vi "LJM logger read program config.vi"(4 "filename":string="expconfig.cfg", 5 "Working Directory":path) -> (0 "error out":errorcluster, 1 "Good Program Config":bool, 2 "Program Configs Out":T1={"Data File Prefix"="", "Scan Rate (Hz)"=0.0, "Graph History"=0, "# Channels"=0, "Disable Scaling"=FALSE, "Max File Size (Bytes)"=0, "Channel Setup"={"Name"=["AIN0", "AIN1", "AIN2", "AIN3", "AIN4", "AIN5", "AIN6", "AIN7", "AIN8", "AIN9", "AIN10", "AIN11", "AIN12", "AIN13", "AIN14", "AIN15"], "", "Scaling Equation"=["y=a", "y=b", "y=c", "y=d", "y=e", "y=f", "y=g", "y=h", "y=i", "y=j", "y=k", "y=l", "y=m", "y=n", "y=o", "y=p"], "", "Graph?"=[TRUE, TRUE, TRUE, TRUE, FALSE, FALSE, FALSE, FALSE, FALSE, FALSE, FALSE, FALSE, FALSE, FALSE, FALSE, FALSE]}, "Interval (ms)"=0, "Write To File"=FALSE, "Log Every n Scans"=0})   [LabVIEW 2026]
uses:
  Common Logger Controls/Program Config Cluster.ctl
  Common Logger Controls/Channel Setup.ctl
  <vilib>/Utility/config.llb/Read Key (String).vi
  <vilib>/Utility/config.llb/Read Key (I32).vi
  <vilib>/Utility/config.llb/Read Key (U32).vi
  <vilib>/Utility/config.llb/Read Key (Double).vi
  <vilib>/Utility/config.llb/Read Key (Boolean).vi
  <vilib>/Utility/config.llb/NI_LVConfig.lvlib
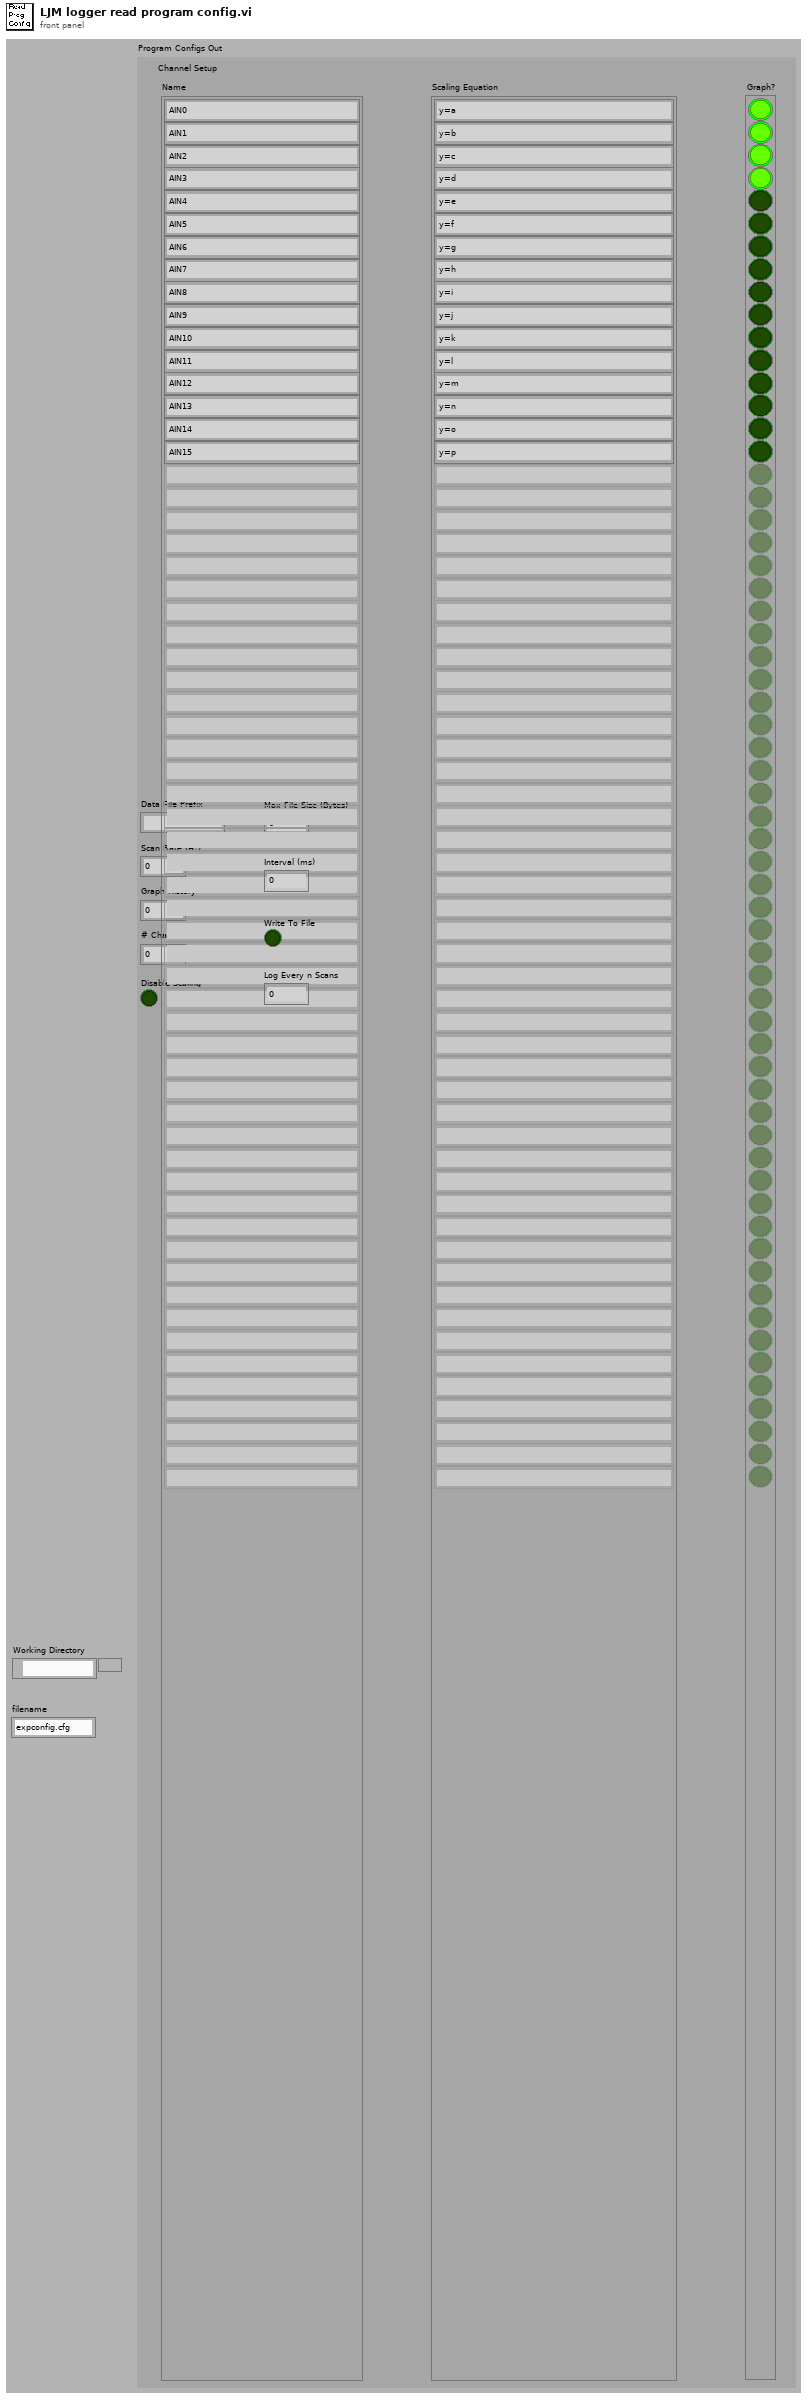
[diagram p1: front panel]
types:
  T1 = typedef "Program Config Cluster.ctl" = cluster{"Data File Prefix":string, "Scan Rate (Hz)":dbl, "Graph History":i32, "# Channels":i32, "Disable Scaling":bool, "Max File Size (Bytes)":i32, "Channel Setup":T2, "Interval (ms)":u32, "Write To File":bool, "Log Every n Scans":i32}
  T2 = typedef "Channel Setup.ctl" = cluster{"Name":string[], string, "Scaling Equation":string[], string, "Graph?":bool[]}
  T3 = typedef "NI_LVConfig.lvlib/Config Data RefNum.ctl" = refnum<k1>
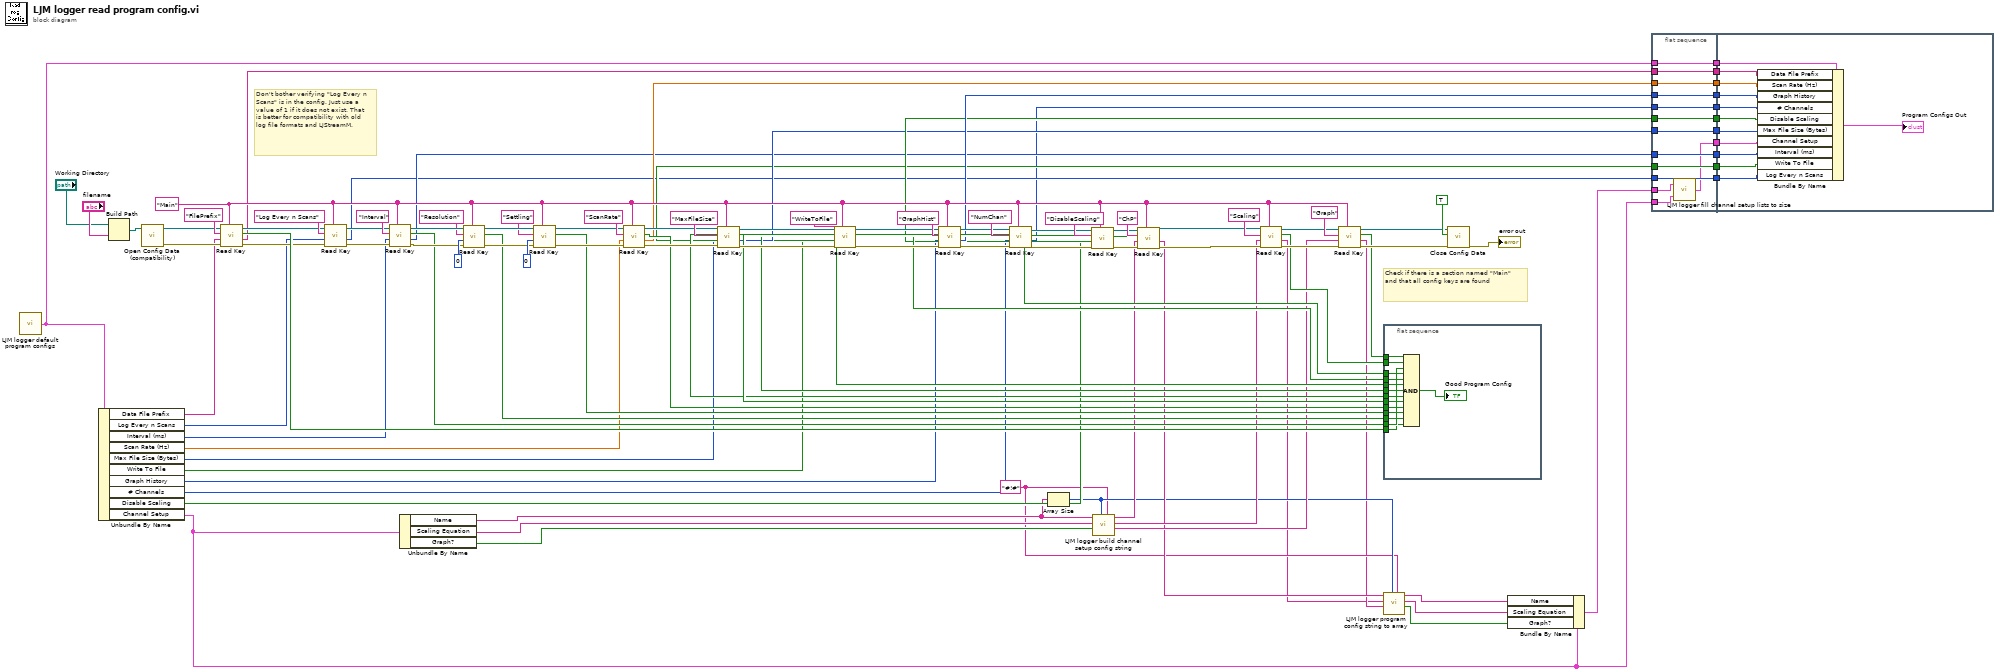
[diagram p0: block diagram]
diagram:
  w6 = "#!#" ("delimiter (#!#)")
  w54 = "Main" ("section")
  # "Don't bother verifying \"Log Every n Scans\" is in the config. Just use a value of 1 if it does not exist. That is better for compatibility with old log file formats and LJStreamM."
  # "Check if there is a section named \"Main\" and that all config keys are found"
  n1 = call "LJM logger default program configs.vi"() -> ("Program Configs"=w10:T1)  [unwired: 1 in]
  n2 = Unbundle By Name(w10) -> ("Data File Prefix"=w35:string, "Log Every n Scans"=w34:i32, "Interval (ms)"=w33:u32, "Scan Rate (Hz)"=w32:dbl, "Max File Size (Bytes)"=w31:i32, "Write To File"=w30:bool, "Graph History"=w29:i32, "# Channels"=w8:i32, "Disable Scaling"=w28:bool, "Channel Setup"=w1:T2)
  n3 = Build Path(base path="Working Directory", name or relative path="filename") -> (appended path=w110:path)
  n4 = call <vilib>:"Open Config Data (compatibility).vi"("configuration file path"=w110) -> ("error out"=w56:errorcluster, "refnum"=w57:T3)  [unwired: 8 in, 1 out]
  n5 = call-poly <vilib>:"Read Key.vi"("section"=w54, "error in (no error)"=w56, "default value"=w35, "key"="FilePrefix", "refnum"=w57) -> ("error out"=w53:errorcluster, "value"=w48:string, "found?"=w69:bool, "refnum out"=w51:T3)  [unwired: 3 in]
  n6 = call-poly <vilib>:"Read Key.vi"("section"=w54, "error in (no error)"=w53, "default value"=w34, "key"="Log Every n Scans", "refnum"=w51) -> ("error out"=w52:errorcluster, "value"=w41:i32, "refnum out"=w50:T3)  [unwired: 3 in, 1 out]
  n7 = call-poly <vilib>:"Read Key.vi"("section"=w54, "error in (no error)"=w52, "default value"=w33, "key"="Interval", "refnum"=w50) -> ("error out"=w85:errorcluster, "value"=w43:u32, "found?"=w68:bool, "refnum out"=w84:T3)  [unwired: 3 in]
  n8 = Unbundle By Name(w1) -> ("Name"=w9:string[], "Scaling Equation"=w26:string[], "Graph?"=w25:bool[])
  n9 = call-poly <vilib>:"Read Key.vi"("section"=w54, "error in (no error)"=w85, "default value"=u8 0 ("Graph History"), "key"="Resolution", "refnum"=w84) -> ("error out"=w87:errorcluster, "found?"=w67:bool, "refnum out"=w86:T3)  [unwired: 3 in, 1 out]
  n10 = call-poly <vilib>:"Read Key.vi"("section"=w54, "error in (no error)"=w87, "default value"=u8 0 ("# Channels"), "key"="Settling", "refnum"=w86) -> ("error out"=w80:errorcluster, "found?"=w66:bool, "refnum out"=w79:T3)  [unwired: 3 in, 1 out]
  n11 = call-poly <vilib>:"Read Key.vi"("section"=w54, "error in (no error)"=w80, "default value"=w32, "key"="ScanRate", "refnum"=w79) -> ("error out"=w76:errorcluster, "value"=w47:dbl, "found?"=w65:bool, "refnum out"=w75:T3)  [unwired: 3 in]
  n12 = call-poly <vilib>:"Read Key.vi"("section"=w54, "error in (no error)"=w76, "default value"=w31, "key"="MaxFileSize", "refnum"=w75) -> ("error out"=w72:errorcluster, "value"=w44:i32, "found?"=w64:bool, "refnum out"=w73:T3)  [unwired: 3 in]
  n13 = call-poly <vilib>:"Read Key.vi"("section"=w54, "error in (no error)"=w72, "default value"=w30, "key"="WriteToFile", "refnum"=w73) -> ("error out"=w70:errorcluster, "value"=w42:bool, "found?"=w63:bool, "refnum out"=w71:T3)  [unwired: 3 in]
  n14 = call-poly <vilib>:"Read Key.vi"("section"=w54, "error in (no error)"=w70, "default value"=w29, "key"="GraphHist", "refnum"=w71) -> ("error out"=w104:errorcluster, "value"=w46:i32, "found?"=w62:bool, "refnum out"=w105:T3)  [unwired: 3 in]
  n15 = call-poly <vilib>:"Read Key.vi"("section"=w54, "error in (no error)"=w104, "default value"=w8, "key"="NumChan", "refnum"=w105) -> ("error out"=w98:errorcluster, "value"=w27:i32, "found?"=w61:bool, "refnum out"=w99:T3)  [unwired: 3 in]
  n16 = Array Size(array=w9) -> (size(s)=w7:i32)
  n17 = call-poly <vilib>:"Read Key.vi"("section"=w54, "error in (no error)"=w98, "default value"=w28, "key"="DisableScaling", "refnum"=w99) -> ("error out"=w97:errorcluster, "value"=w45:bool, "found?"=w60:bool, "refnum out"=w96:T3)  [unwired: 3 in]
  n18 = call "LJM logger build channel setup config string.vi"("delimiter (#!#)"=w6, "Max Num Elements"=w7, "Bool list"=w25, "String list 2"=w26, "String list 1"=w9) -> ("Bool formatted"=w36:string, "String 2 formatted"=w37:string, "String 1 formatted"=w38:string)  [unwired: 3 in, 1 out]
  n19 = call-poly <vilib>:"Read Key.vi"("section"=w54, "error in (no error)"=w97, "default value"=w38, "key"="ChP", "refnum"=w96) -> ("error out"=w39:errorcluster, "value"=w12:string, "found?"=w49:bool, "refnum out"=w40:T3)  [unwired: 3 in]
  n20 = call-poly <vilib>:"Read Key.vi"("section"=w54, "error in (no error)"=w39, "default value"=w37, "key"="Scaling", "refnum"=w40) -> ("error out"=w94:errorcluster, "value"=w2:string, "found?"=w59:bool, "refnum out"=w91:T3)  [unwired: 3 in]
  n21 = call-poly <vilib>:"Read Key.vi"("section"=w54, "error in (no error)"=w94, "default value"=w36, "key"="Graph", "refnum"=w91) -> ("error out"=w93:errorcluster, "value"=w5:string, "found?"=w58:bool, "refnum out"=w92:T3)  [unwired: 3 in]
  n22 = flat-sequence {
    tunnel: w69 -> [w112]
    tunnel: w68 -> [w125]
    tunnel: w67 -> [w124]
    tunnel: w66 -> [w123]
    tunnel: w65 -> [w122]
    tunnel: w64 -> [w121]
    tunnel: w63 -> [w120]
    tunnel: w62 -> [w119]
    tunnel: w61 -> [w118]
    tunnel: w60 -> [w117]
    tunnel: w49 -> [w116]
    tunnel: w59 -> [w115]
    tunnel: w58 -> [w114]
    frame #0 {
      n23 = Compound Arithmetic op=AND(w114, w115, w116, w117, w118, w119, w120, w121, w122, w123, w124, w125, w112) -> (→"Good Program Config":bool)
    }
  }
  n24 = call "LJM logger program config string to array.vi"("Delimiter (#!#)"=w6, "Max Num Elements"=w7, "Bool Config String In"=w5, "String Config String In 2"=w2, "String Config String In"=w12) -> ("Bool Config Array Out"=w4:bool[], "String Config Array Out 2"=w3:string[], "String Config Array Out"=w11:string[])  [unwired: 3 in, 1 out]
  n25 = call <vilib>:"Close Config Data.vi"("error in (no error)"=w93, "write file if changed (T)"=TRUE ("write configuration file? (F)"), "refnum"=w92) -> ("error out"=→"error out":errorcluster)  [unwired: 7 in, 1 out]
  n26 = Bundle By Name(cluster=w1, "Name"=w11, "Scaling Equation"=w3, "Graph?"=w4) -> (w13:T2)
  n27 = flat-sequence {
    tunnel: w10 -> [w129]
    tunnel: w27 -> [w130]
    tunnel: w41 -> [w131]
    tunnel: w42 -> [w132]
    tunnel: w43 -> [w133]
    tunnel: w44 -> [w134]
    tunnel: w45 -> [w135]
    tunnel: w46 -> [w136]
    tunnel: w47 -> [w137]
    tunnel: w48 -> [w138]
    tunnel: [w138] -> w24
    tunnel: [w137] -> w23
    tunnel: [w136] -> w22
    tunnel: [w135] -> w21
    tunnel: [w134] -> w20
    tunnel: [w133] -> w19
    tunnel: [w132] -> w18
    tunnel: [w131] -> w17
    tunnel: [w130] -> w16
    tunnel: [w129] -> w15
    tunnel: [w128] -> w14
    tunnel: w1 -> [w127]
    tunnel: w13 -> [w126]
    tunnel: w24 -> [w150]
    tunnel: w23 -> [w148]
    tunnel: w22 -> [w147]
    tunnel: w21 -> [w146]
    tunnel: w20 -> [w145]
    tunnel: w19 -> [w144]
    tunnel: w18 -> [w143]
    tunnel: w17 -> [w142]
    tunnel: w16 -> [w141]
    tunnel: w15 -> [w140]
    tunnel: w14 -> [w139]
    frame #0 {
      n28 = call "LJM logger fill channel setup lists to size.vi"("Default Channel Setup"=w127, "Channel Setup In"=w126) -> ("Channel Setup Out"=w128:T2)
    }
    frame #1 {
      n29 = Bundle By Name(cluster=w140, "Data File Prefix"=w150, "Scan Rate (Hz)"=w148, "Graph History"=w147, "# Channels"=w141, "Disable Scaling"=w146, "Max File Size (Bytes)"=w145, "Channel Setup"=w139, "Interval (ms)"=w144, "Write To File"=w143, "Log Every n Scans"=w142) -> (→"Program Configs Out":T1)
    }
  }
